vi "Set Length.vi"(10 "Max String Length":i32, 11 "Input":string) -> (3 "Output":string)   [LabVIEW 2010]
panel:
  # "This VI will keep the output string length to that set by the Max String Length input by deleting from the beginning of the string."
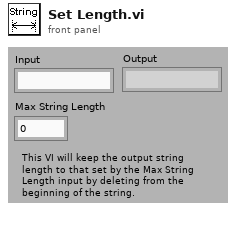
[diagram p1: front panel]
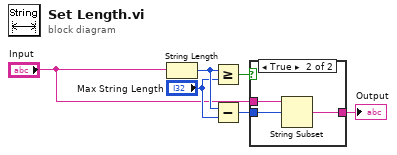
[diagram p0: block diagram]
diagram:
  n1 = String Length(string="Input") -> (length=w5:i32)
  n2 = Greater Or Equal?(x=w5, y="Max String Length") -> (x >= y?=w6:bool)
  n3 = Subtract(x=w5, y="Max String Length") -> (x-y=w3:i32)
  n4 = case shown="True" w6 {
    tunnel: [w7 w10] -> w1
    tunnel: w3 -> [_ w9]
    tunnel: "Input" -> [w7 w8]
    frame False {
    }
    frame True {
      n5 = String Subset(string=w8, offset (0)=w9) -> (substring=w10:string)  [unwired: 1 out]
    }
  }
  "Output" <- w1
